vi "System Status Management Core.vi"(11 "CIFPluginManager in":refnum<class "CIFPluginManager.lvclass">) -> (0 "error out":errorcluster)   [LabVIEW 2021, in "CIFPluginManager.lvclass"]
uses:
  CIFPluginManager.lvclass
  CIFPluginManager.lvclass/CIFPluginManager.ctl
  gRPC/CIF_Manager_server/RPC Service/Manager/Manager.lvclass
  C:/Program Files/National Instruments/LabVIEW 2021/vi.lib/gRPC/LabVIEW gRPC Servicer/ServiceBase/ServiceBase.lvclass
  gRPC/CIF_Manager_server/RPC Service/Manager/Manager.lvclass/Manager.ctl
  gRPC/CIF_Manager_server/RPC Messages/cif_manager_SystemStatus.ctl
  gRPC/CIF_Manager_server/RPC Messages/cif_manager_ClockConversionArray.ctl
  gRPC/CIF_Manager_server/RPC Messages/cif_manager_ClockConversion.ctl
  gRPC/CIF_Manager_server/RPC Messages/cif_manager_TimePair.ctl
  gRPC/CIF_Manager_server/RPC Messages/Get cif_manager_PluginStatus.vi
  gRPC/CIF_Manager_server/RPC Messages/Set cif_manager_SystemStatus.vi
  gRPC/CIF_Manager_server/RPC Messages/Get cif_manager_PluginStatus.vi/2ed25e12-861d-4677-8ead-ace2906b2041.vi
  gRPC/CIF_Manager_server/RPC Messages/FlatToRichcif_manager_PluginStatus.vi
  gRPC/CIF_Manager_server/RPC Messages/Set cif_manager_SystemStatus.vi/dcc74a39-081a-4bdd-860b-8ed792803c96.vi
  gRPC/CIF_Manager_server/RPC Messages/RichToFlatcif_manager_SystemStatus.vi
  <vilib>/gRPC/LabVIEW gRPC Library/Shared/TranslateGrpcError.vi
  gRPC/CIF_Manager_server/RPC Messages/FlatToRichcif_manager_PluginName.vi
  gRPC/CIF_Manager_server/RPC Messages/FlatToRichcif_plugincore_StatusData.vi
  gRPC/CIF_Manager_server/RPC Messages/FlatToRichcif_channelcore_Channels.vi
  gRPC/CIF_Manager_server/RPC Messages/RichToFlatcif_manager_ClockConversionArray.vi
  gRPC/CIF_Manager_server/RPC Messages/FlatToRichcif_plugincore_TimingStatistics.vi
  gRPC/CIF_Manager_server/RPC Messages/FlatToRichcif_plugincore_FifoStatistics.vi
  gRPC/CIF_Manager_server/RPC Messages/FlatToRichcif_plugincore_Error.vi
  gRPC/CIF_Manager_server/RPC Messages/FlatToRichcif_plugincore_MonitorDoubles.vi
  gRPC/CIF_Manager_server/RPC Messages/FlatToRichcif_plugincore_MonitorU64.vi
  gRPC/CIF_Manager_server/RPC Messages/FlatToRichcif_plugincore_MonitorI64.vi
  gRPC/CIF_Manager_server/RPC Messages/FlatToRichcif_channelcore_Channel.vi
  gRPC/CIF_Manager_server/RPC Messages/RichToFlatcif_manager_ClockConversion.vi
  gRPC/CIF_Manager_server/RPC Messages/FlatToRichcif_common_TimingStats.vi
  gRPC/CIF_Manager_server/RPC Messages/RichToFlatcif_manager_TimePair.vi
  <vilib>/gRPC/LabVIEW gRPC Library/Server API/Server/Get Server DLL Path.vi
  <vilib>/Utility/error.llb/Error Cluster From Error Code.vi
  <vilib>/gRPC/LabVIEW gRPC Library/Server API/Message Requests/Complete Call.vi
  CIFUtilities/CIFLogs/CIFLogs.lvlib
  gRPC/CIF_Manager_server/CIF_Manager_server.lvlib
  <vilib>/CIF Foundation/CIF Utilities/Time/Time_CIF_U.lvlib
  gRPC/CIF_Manager_Client_Wrapper/CIFManagerClientWrapper.lvlib
  D:/dev/CIF-LVCore/src/CIFPluginManager/CIFPluginManager/gRPC/CIF_Manager_server/RPC Service/Manager/Manager.lvclass
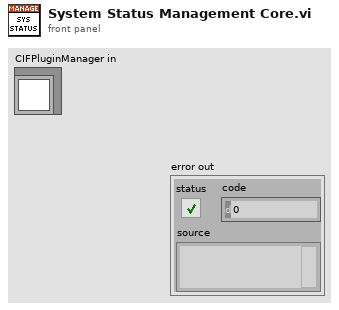
[diagram p1: front panel]
types:
  T1 = typedef "CIF_Manager_server.lvlib/Manager.lvclass/Server gRPC UEs.ctl" = cluster{"Manager LoadPlugin gRPC UE":refnum<user-event>, "Manager RegisterPlugin gRPC UE":refnum<user-event>, "Manager UnregisterPlugin gRPC UE":refnum<user-event>, "Manager QueryPluginTypes gRPC UE":refnum<user-event>, "Manager AbortPlugin gRPC UE":refnum<user-event>, "Manager UnloadAllPlugins gRPC UE":refnum<user-event>, "Manager Destroy gRPC UE":refnum<user-event>, "Manager Ping gRPC UE":refnum<user-event>, "Manager QueryErrors gRPC UE":refnum<user-event>, "Manager QueryConfig gRPC UE":refnum<user-event>, "Manager QueryInfo gRPC UE":refnum<user-event>, "Manager ResetErrorIndex gRPC UE":refnum<user-event>, "Manager ResetConfigIndex gRPC UE":refnum<user-event>, "Manager ResetInfoIndex gRPC UE":refnum<user-event>, "Manager QueryPluginInfo gRPC UE":refnum<user-event>, "Manager QueryPlugin gRPC UE":refnum<user-event>, "Manager QuerySystemStatus gRPC UE":refnum<user-event>, "Manager UpdateClock gRPC UE":refnum<user-event>, "Manager CreateOrch gRPC UE":refnum<user-event>, "Manager QueryClockStatus gRPC UE":refnum<user-event>, "Manager QueryAllChannels gRPC UE":refnum<user-event>, "Manager RegisterPluginLoader gRPC UE":refnum<user-event>, "Manager UnregisterPluginLoader gRPC UE":refnum<user-event>, "Manager CreatePluginLoader gRPC UE":refnum<user-event>, "Manager DestroyPluginLoader gRPC UE":refnum<user-event>, "Manager QueryPluginLoaders gRPC UE":refnum<user-event>}
  T2 = typedef "CIF_Manager_server.lvlib/cif_manager_SystemStatus.ctl" = cluster{"clock_conversion_array":T3}
  T3 = typedef "CIF_Manager_server.lvlib/cif_manager_ClockConversionArray.ctl" = cluster{"clock_conversions":T4[]}
  T4 = typedef "CIF_Manager_server.lvlib/cif_manager_ClockConversion.ctl" = cluster{"clock_id":u32, "last_reset":i64, "slope":dbl, "offset_pair":T5, "clock_name":string}
  T5 = typedef "CIF_Manager_server.lvlib/cif_manager_TimePair.ctl" = cluster{"system_time":i64, "external_time":i64}
  T6 = typedef "grpc-lvsupport-release.lvlib/grpcId.ctl" = u64
  T7 = typedef "CIF_Manager_server.lvlib/cif_manager_PluginStatus.ctl" = cluster{"pluginname":T8, "status":T9, "channels":T18}
  T8 = typedef "CIF_Manager_server.lvlib/cif_manager_PluginName.ctl" = cluster{"plugin_name":string}
  T9 = typedef "CIF_Manager_server.lvlib/cif_plugincore_StatusData.ctl" = cluster{"state":T10, "timing_statistics":T11, "fifo_statistics":T13, "error":T14, "monitor_doubles":T15, "monitor_u64s":T16, "monitor_i64s":T17}
  T10 = typedef "CIF_Manager_server.lvlib/cif_plugincore_StatusData_PluginState.ctl" = enum32{"PLUGINSTATE_UNKNOWN", "PLUGINSTATE_CREATING", "PLUGINSTATE_LISTENING", "PLUGINSTATE_RUNNING", "PLUGINSTATE_CLEANINGUP", "PLUGINSTATE_DESTROYING"}
  T11 = typedef "CIF_Manager_server.lvlib/cif_plugincore_TimingStatistics.ctl" = cluster{"period":T12, "wake_error":T12, "execute":T12, "housekeep":T12, "idle":T12, "cleanup":T12, "custom_1":T12, "custom_2":T12}
  T12 = typedef "CIF_Manager_server.lvlib/cif_common_TimingStats.ctl" = cluster{"max":i64, "min":i64, "avg":dbl}
  T13 = typedef "CIF_Manager_server.lvlib/cif_plugincore_FifoStatistics.ctl" = cluster{"from_t0":T12, "from_previous_plugin":T12, "output_error":T12}
  T14 = typedef "CIF_Manager_server.lvlib/cif_plugincore_Error.ctl" = cluster{"status":bool, "code":i32}
  T15 = typedef "CIF_Manager_server.lvlib/cif_plugincore_MonitorDoubles.ctl" = cluster{"double_1":dbl, "double_2":dbl, "double_3":dbl, "double_4":dbl}
  T16 = typedef "CIF_Manager_server.lvlib/cif_plugincore_MonitorU64.ctl" = cluster{"u64_1":u64, "u64_2":u64, "u64_3":u64, "u64_4":u64}
  T17 = typedef "CIF_Manager_server.lvlib/cif_plugincore_MonitorI64.ctl" = cluster{"i64_1":i64, "i64_2":i64, "i64_3":i64, "i64_4":i64}
  T18 = typedef "CIF_Manager_server.lvlib/cif_channelcore_Channels.ctl" = cluster{"channels":T19[]}
  T19 = typedef "CIF_Manager_server.lvlib/cif_channelcore_Channel.ctl" = cluster{"name":string, "direction":T20, "type":string, "custom_config":u8[], "connected":bool, "connected_name":string, "forced":bool, "channel_pattern":T21}
  T20 = typedef "CIF_Manager_server.lvlib/cif_channelcore_ChannelDirection.ctl" = enum32{"CHANNELDIRECTION_UNKNOWN", "CHANNELDIRECTION_PUBLISHER", "CHANNELDIRECTION_SUBSCRIBER"}
  T21 = typedef "CIF_Manager_server.lvlib/cif_channelcore_ChannelPattern.ctl" = enum32{"CHANNELPATTERN_UNKNOWN", "CHANNELPATTERN_TAG", "CHANNELPATTERN_FIFO", "CHANNELPATTERN_MULTIFIFO", "CHANNELPATTERN_BACKPRESSUREFIFO"}
  T22 = typedef "Time_CIF_U.lvlib/Clock History Map.ctl" = map{u8, T23}
  T23 = typedef "Time_CIF_U.lvlib/Clock History.ctl" = cluster{"System Clock":i64[], "External Clock":i64[], "Last Reset Time":i64, "slope":dbl, "1/slope":dbl, "Offset Pair":T24, "Name":string}
  T24 = typedef "Time_CIF_U.lvlib/Timestamp Pair.ctl" = cluster{"System Time":i64, "External Time":i64}
  T25 = typedef "Time_CIF_U.lvlib/Clock Conversion.ctl" = cluster{"ClockID":u8, "Last Reset":i64, "Offset Pair":T24, "Slope":dbl, "1/Slope":dbl, "Name":string}
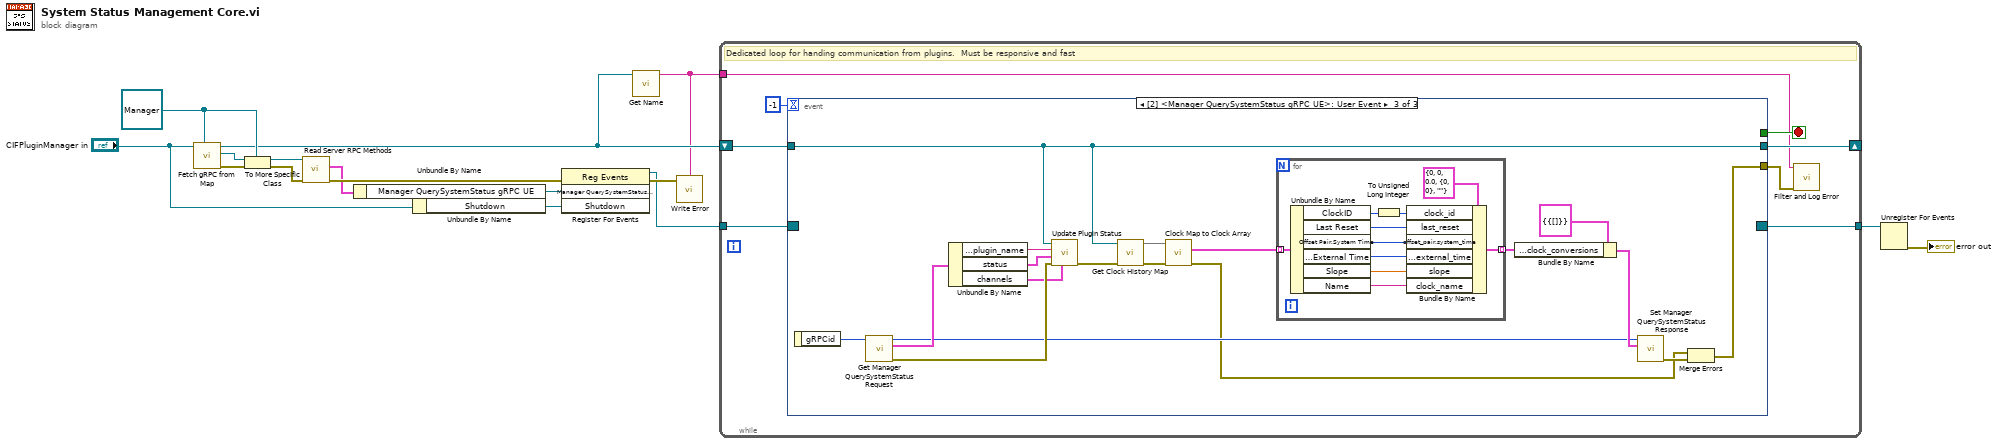
[diagram p0: block diagram]
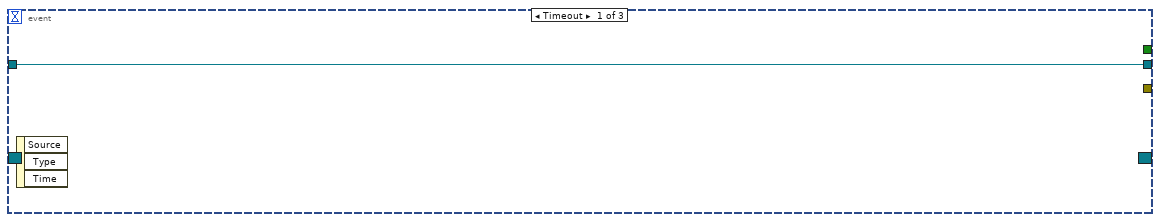
[diagram p2: hidden frame]
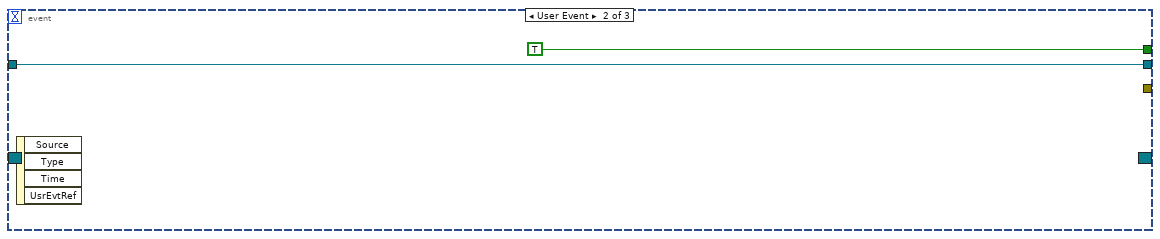
[diagram p3: hidden frame]
diagram:
  w13 = refnum<class "Manager.lvclass"> refnum ("CIF_Manager_server.lvlib:Manager.lvclass")
  n1 = call "Fetch gRPC from Map.vi"("gRPC Server Class type"=w13, "Plugin Manager in"="CIFPluginManager in") -> ("error out"=w12:errorcluster, "gRPC Server Class out"=w14:refnum<class "ServiceBase.lvclass">, "Plugin Manager out"=w2:refnum<class "CIFPluginManager.lvclass">)  [unwired: 7 in]
  n2 = To More Specific Class(target class=w13, reference=w14, error in=w12) -> (specific class reference=w10:refnum<class "Manager.lvclass">, error out=w11:errorcluster)
  n3 = call "Read Server RPC Methods.vi"("error in (no error)"=w11, "gRPC service in"=w10) -> ("error out"=w5:errorcluster, "Server RPC Methods"=w4:T1)  [unwired: 7 in, 1 out]
  n4 = Unbundle By Name(w4) -> ("Manager QuerySystemStatus gRPC UE"=w3:refnum<user-event>)
  n5 = Unbundle By Name("CIFPluginManager in") -> ("Shutdown"=w9:refnum<user-event>)
  n6 = register-events(error in=w5, w3, w9) -> (reference out=w6:refnum<event-registration>, error out=w7:errorcluster)  [unwired: 1 in]
  n7 = call "Get Name.vi"("CIFPluginManager in"=w2) -> ("Name"=w1:string)  [unwired: 10 in]
  n8 = call "Write Error.vi"("error in (no error)"=w7, "Plugin Name"=w1) -> ()  [unwired: 2 in, 1 out]
  n9 = while {
    tunnel: w6 -> [w24]
    shift-right: [w19] -> _
    shift-left: w2 -> [w23]
    tunnel: [w20] -> w15
    tunnel: w1 -> [w17]
    stop <- w21 stop-if-true
    # "Dedicated loop for handing communication from plugins.  Must be responsive and fast"
    n10 = event shown="[2] <Manager QuerySystemStatus gRPC UE>: User Event" {
      selector: w24 -> [_ _ _]
      dyn-events: [_ _ _] -> w20
      timeout: -1 -> [_ _ _]
      tunnel: w23 -> [w25 w26 w29]
      tunnel: [_ TRUE _] -> w21
      tunnel: [_ _ w34] -> w18
      tunnel: [w25 w26 w29] -> w19
      event Timeout {
        n11 = event-data() -> ()  [unwired: 1 in, 3 out]
      }
      event User Event {
        n12 = event-data() -> ()  [unwired: 1 in, 4 out]
      }
      event User Event {
        n13 = event-data() -> ("gRPCid"=w35:T6)  [unwired: 1 in]
        n14 = call "Get Manager QuerySystemStatus Request.vi"("gRPCid"=w35) -> ("error out"=w44:errorcluster, "Message Data"=w41:T7, "gRPCid out"=w37:T6)  [unwired: 8 in]
        n15 = Unbundle By Name(w41) -> ("pluginname.plugin_name"=w42:string, "status"=w43:T9, "channels"=w28:T18)
        n16 = call "Update Plugin Status.vi"("channels"=w28, "error in (no error)"=w44, "Status"=w43, "Plugin Name"=w42, "Launcher in"=w29) -> ("error out"=w32:errorcluster)  [unwired: 6 in]
        n17 = call "Get Clock History Map.vi"("error in (no error)"=w32, "CIFPluginManager in"=w29) -> ("error out"=w31:errorcluster, "Clock History Map"=w33:T22)  [unwired: 8 in]
        n18 = call <vilib>:"Clock Map to Clock Array.vi"("error in (no error)"=w31, "Clock History Map in"=w33) -> ("error out"=w30:errorcluster, "Clock Conversion Array"=w45:T25[])  [unwired: 7 in, 1 out]
        n19 = for {
          tunnel: w45 -> [w54] mode=indexing
          tunnel: [w46] -> w39 mode=indexing
          n20 = Unbundle By Name(w54) -> ("ClockID"=w53:u8, "Last Reset"=w47:i64, "Offset Pair.System Time"=w48:i64, "Offset Pair.External Time"=w49:i64, "Slope"=w50:dbl, "Name"=w51:string)
          n21 = To Unsigned Long Integer(number=w53) -> (unsigned 32bit integer=w52:u32)
          n22 = Bundle By Name(cluster=T4 {"clock_id"=0, "last_reset"=0, "slope"=0.0, "offset_pair"={"system_time"=0, "external_time"=0}, "clock_name"=""} ("cif_manager_ClockConversion"), "clock_id"=w52, "last_reset"=w47, "offset_pair.system_time"=w48, "offset_pair.external_time"=w49, "slope"=w50, "clock_name"=w51) -> (w46:T4)
        }
        n23 = Bundle By Name(cluster=T2 {"clock_conversion_array"={"clock_conversions"=[]}} ("Message Data"), "clock_conversion_array.clock_conversions"=w39) -> (w40:T2)
        n24 = call "Set Manager QuerySystemStatus Response.vi"("Message Data"=w40, "gRPCid in"=w37) -> ("error out"=w38:errorcluster)  [unwired: 9 in]
        n25 = Merge Errors(w30, w38) -> (w34:errorcluster)
      }
    }
    n26 = call "Filter and Log Error.vi"("error In"=w18, "Name"=w17) -> ()  [unwired: 10 in]
  }
  n27 = Unregister For Events(event registration refnum=w15) -> (error out=→"error out":errorcluster)  [unwired: 1 in]
